vi "pinout-settings.vi"(7 "LabVIEW Web Service Request":refnum<class "Web Request.lvclass">, 9 "outdoor-temp-pin":u8=2, 10 "main_fan_pin":u8=9, 11 "main_light_pin":u8=8) -> ()   [LabVIEW 2023]
uses:
  <vilib>/wsapi/Web Request.lvclass
  PinoutSettings.vi
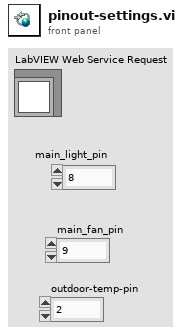
[diagram p1: front panel]
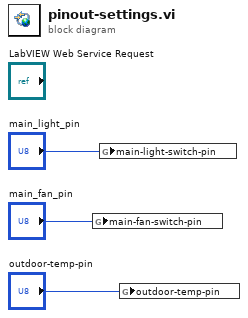
[diagram p0: block diagram]
diagram:
  n1 = global write "PinoutSettings.vi" "main-fan-switch-pin"("main_fan_pin") -> ()
  n2 = global write "PinoutSettings.vi" "main-light-switch-pin"("main_light_pin") -> ()
  n3 = global write "PinoutSettings.vi" "outdoor-temp-pin"("outdoor-temp-pin") -> ()
